vi "STED Control V4.vi"() -> ()   [LabVIEW 2014]
uses:
  Type Defs/Image Acquisition Parameters.ctl
  Laser Controls.ctl
  Detectors.ctl
  Stage Control.ctl
  Focus Control.ctl
  FPGA-7842R-Reference.ctl
  Scan Parameters.ctl
  Manual Controls V2.ctl
  XY_Stage/StageStates.ctl
  <vilib>/Utility/miscctls.llb/LVRectTypeDef.ctl
panel:
  in  "Tab Control":T1(tab)
  in  "SLM":bool
  in  "Timing":bool
  in  "Focus Control":T2
  in  "Stage Control":T3={"Halt"=FALSE, "Home"=FALSE, "Down Stage"=FALSE, "Right Stage"=FALSE, "Up Stage"=FALSE, "Left Stage"=FALSE, "Mode"=enum."Joystick", "X Position"=1.0, "Y Position"=1.0, "Step Size (um)"=enum."1", "Velocity"=enum."Low"} {"Y Position" min=1.0 max=24.0; "X Position" min=1.0 max=24.0}
  out "Channel 6":sgl[][](graph)
  out "Channel 5":sgl[][](graph)
  out "Channel 4":sgl[][](graph)
  out "Channel 3":sgl[][](graph)
  out "Channel 2":sgl[][](graph)
  in  "Dual Screens":bool=TRUE
  in  "Detectors":T4
  in  "Laser Controls":T5 {"590 Power (V)" scale=0.0..3.0; "STED Power (V)" scale=0.0..5.0}
  in  "Save File Path":path
  in  "Capture":bool
  out "Channel 1":sgl[][](graph)
  in  "Image Acquisition Parameters":T6={"Scan Type"=enum."Beam Scanning", "Scan Mode"=enum."XY", "Fast Axis Frequency (Hz)"=16110.0, "Image Format"=256, "Line Accumulations"=100, "Frames Per Capture"=1, "Frames Accumulations"=1, "Image Dimension (um)"=[15.0, 15.0], "Number of Z Steps"=1, "Z Steps Size (um)"=1.0, "Pixel Size (nm)"=[58.59375, 58.59375]} {"Z Steps Size (um)" min=0.0; "Number of Z Steps" min=1; "Frames Accumulations" min=1; "Frames Per Capture" min=1; "Line Accumulations" min=1; "Image Format" items=["64 x 64"=64, "128 x 128"=128, "256 x 256"=256, "512 x 512"=512, "1024 x 1024"=1024, "2048 x 2048"=2048]}
  in  "Live":bool
  in  "Exit":bool
  # "XY"
  # "Z"
  # "Length"
  # "Height"
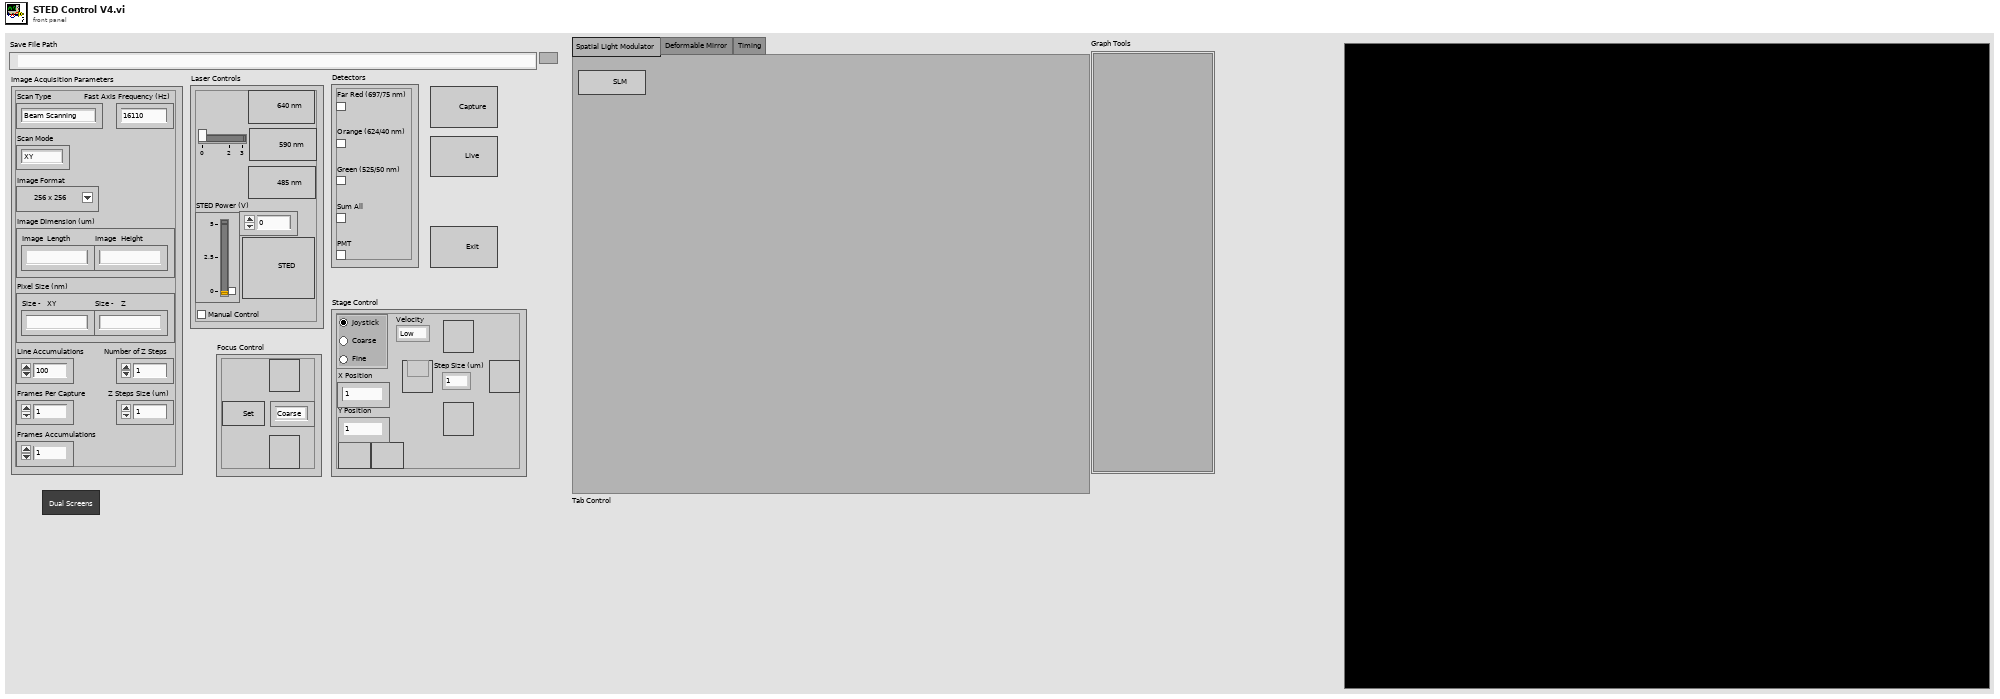
[diagram p1: front panel]
types:
  T1 = enum32{"Spatial Light Modulator", "Deformable Mirror", "Timing"}
  T2 = typedef "Focus Control.ctl" = cluster{"ZoomUp":bool, "ZoomDown":bool, "ZoomStepI16":enum16{"Coarse", "Medium", "Fine"}, "SetZoom":bool}
  T3 = typedef "Stage Control.ctl" = cluster{"Halt":bool, "Home":bool, "Down Stage":bool, "Right Stage":bool, "Up Stage":bool, "Left Stage":bool, "Mode":enum32{"Joystick", "Coarse", "Fine"}, "X Position":dbl, "Y Position":dbl, "Step Size (um)":enum16{"1", "2", "5", "10", "15", "20", "50", "100", "500"}, "Velocity":enum16{"Low", "Medium", "High"}}
  T4 = typedef "Detectors.ctl" = cluster{"PMT":bool, "Far Red (697/75 nm)":bool, "Orange (624/40 nm)":bool, "Green (525/50 nm)":bool, "Sum All":bool}
  T5 = typedef "Laser Controls.ctl" = cluster{"STED Power (V)":dbl, "590 Power (V)":dbl, "STED":bool, "640 nm":bool, "590 nm":bool, "485 nm":bool, "Manual Control":bool}
  T6 = typedef "Image Acquisition Parameters.ctl" = cluster{"Scan Type":enum16{"Sample Scanning", "Beam Scanning"}, "Scan Mode":enum16{"XY", "XZ", "YZ", "XYZ"}, "Fast Axis Frequency (Hz)":dbl, "Image Format":u16, "Line Accumulations":u16, "Frames Per Capture":u16, "Frames Accumulations":u16, "Image Dimension (um)":dbl[], "Number of Z Steps":u8, "Z Steps Size (um)":dbl, "Pixel Size (nm)":dbl[]}
  T7 = typedef "Manual Controls V2.ctl" = cluster{"Galvo 1 Position (I16)":i16, "Galvo 2 Position (I16)":i16, "X Axis Voltage (I16)":i16, "Y Axis Voltage (I16)":i16, "Z Axis Voltage (I16)":i16, "Res Mirror Amp (I16)":i16, "Res Mirror Mute":bool}
  T8 = typedef "Scan Parameters.ctl" = cluster{"Fast_Ax_Amp_V":dbl, "Fast_Ax_Off_V":dbl, "Slow_Ax_Amp_V":dbl, "Slow_Ax_Off_V ":dbl, "Slow_Ax_Max_V_VperS":dbl, "Slow_Ax1_Del25ns":i32, "Slow_Ax2_Del25ns":i32, "Stage_X_Off_V":dbl, "Stage_Y_Off_V":dbl, "Stage_Z_Off_V":dbl, "Galvo1_Off_V":dbl, "Galvo2_Off_V":dbl, "Last_Scan_Mode":enum16{"XY", "XZ", "YZ", "XYZ"}, "Current_Scan_Mode":enum16{"XY", "XZ", "YZ", "XYZ"}, "Fly_Back_Lines":u16, "Linear_Ramp_End":u32, "Z_Step_I16":i16, "Z_Start_I16":i16, "Laser_States _U32":u32, "590_Voltage_I16":i16, "775_AOM_Volt_I16":i16, "Blanking OFF":bool, "Unused_Axis_I16":i16}
  T9 = typedef "FPGA-7842R-Reference.ctl" = enum16{"Stage Control", "Laser Control", "Unused Axis I16", "Exit", "Set Res Mirror", "Set Galvo", "Default", "Close FPGA", "Stop Waveforms", "Start Waveforms", "Initialize"}
  T10 = typedef "StageStates.ctl" = enum16{"POSITION", "MVR", "MOVE", "HALT", "ONTARGET", "ERROR", "EXIT", "HOME", "ZEROPOS", "NANOPOS", "QUIT", "SERVO", "JOYSTICK", "ANALOG"}
  T11 = typedef "LVRectTypeDef.ctl" = cluster{"Left":i16, "Top":i16, "Right":i16, "Bottom":i16}
  T12 = enum32{"Invalid", "Standard", "Closed", "Hidden", "Minimized", "Maximized"}
  T13 = cluster{"Halt":bool, "Home":bool, "Down Stage":bool, "Right Stage":bool, "Up Stage":bool, "Left Stage":bool, "Mode":bool, "X Position":bool, "Y Position":bool, "Step Size (um)":bool, "Velocity":bool}
  T14 = enum16{"1", "2", "5", "10", "15", "20", "50", "100", "500"}
  T15 = typedef "Scanning Conversions.ctl" = cluster{"Stage X Axis (Volts/um)":dbl, "Stage Y Axis (Volts/um)":dbl, "Stage Z Axis (Volts/um)":dbl}
  T16 = typedef "LVAllMonitorsDisplayTypeDef.ctl" = cluster{"Bounds":cluster{"Left":i16, "Top":i16, "Right":i16, "Bottom":i16}, "Depth":i16}[]
  T17 = cluster{"Bounds":cluster{"Left":i16, "Top":i16, "Right":i16, "Bottom":i16}, "Depth":i16}
  T18 = cluster{"Scan Type":bool, "Scan Mode":bool, "Fast Axis Frequency (Hz)":bool, "Image Format":bool, "Line Accumulations":bool, "Frames Per Capture":bool, "Frames Accumulations":bool, "Image Dimension (um)":bool[], "Number of Z Steps":bool, "Z Steps Size (um)":bool, "Pixel Size (nm)":bool[]}
  T19 = typedef "IMAQ Image.ctl" = refnum<image>
  T20 = typedef "Waveform Data.ctl" = cluster{"Waveform Scan Parameters":cluster{"Scanning Mode":u8, "Fast Axis WF Length (Elements)":i32, "Fast Axis Sample Period (Ticks)":u32, "Slow Axis 1 WF Length (Elements)":i32, "Slow Axis 1 Sample Period (Ticks)":u32, "Slow Axis 1 Delay (25 ns) Steps":i32, "Slow Axis 2 WFLength (Elements)":i32, "Slow Axis 2 Sample Period (Ticks)":u32, "Slow Axis 2 Delay (25 ns) Steps":i32}, "Fast Axis Waveform":dbl[], "Slow Axis 1 Waveform":dbl[], "Slow Axis 2 Waveform":dbl[]}
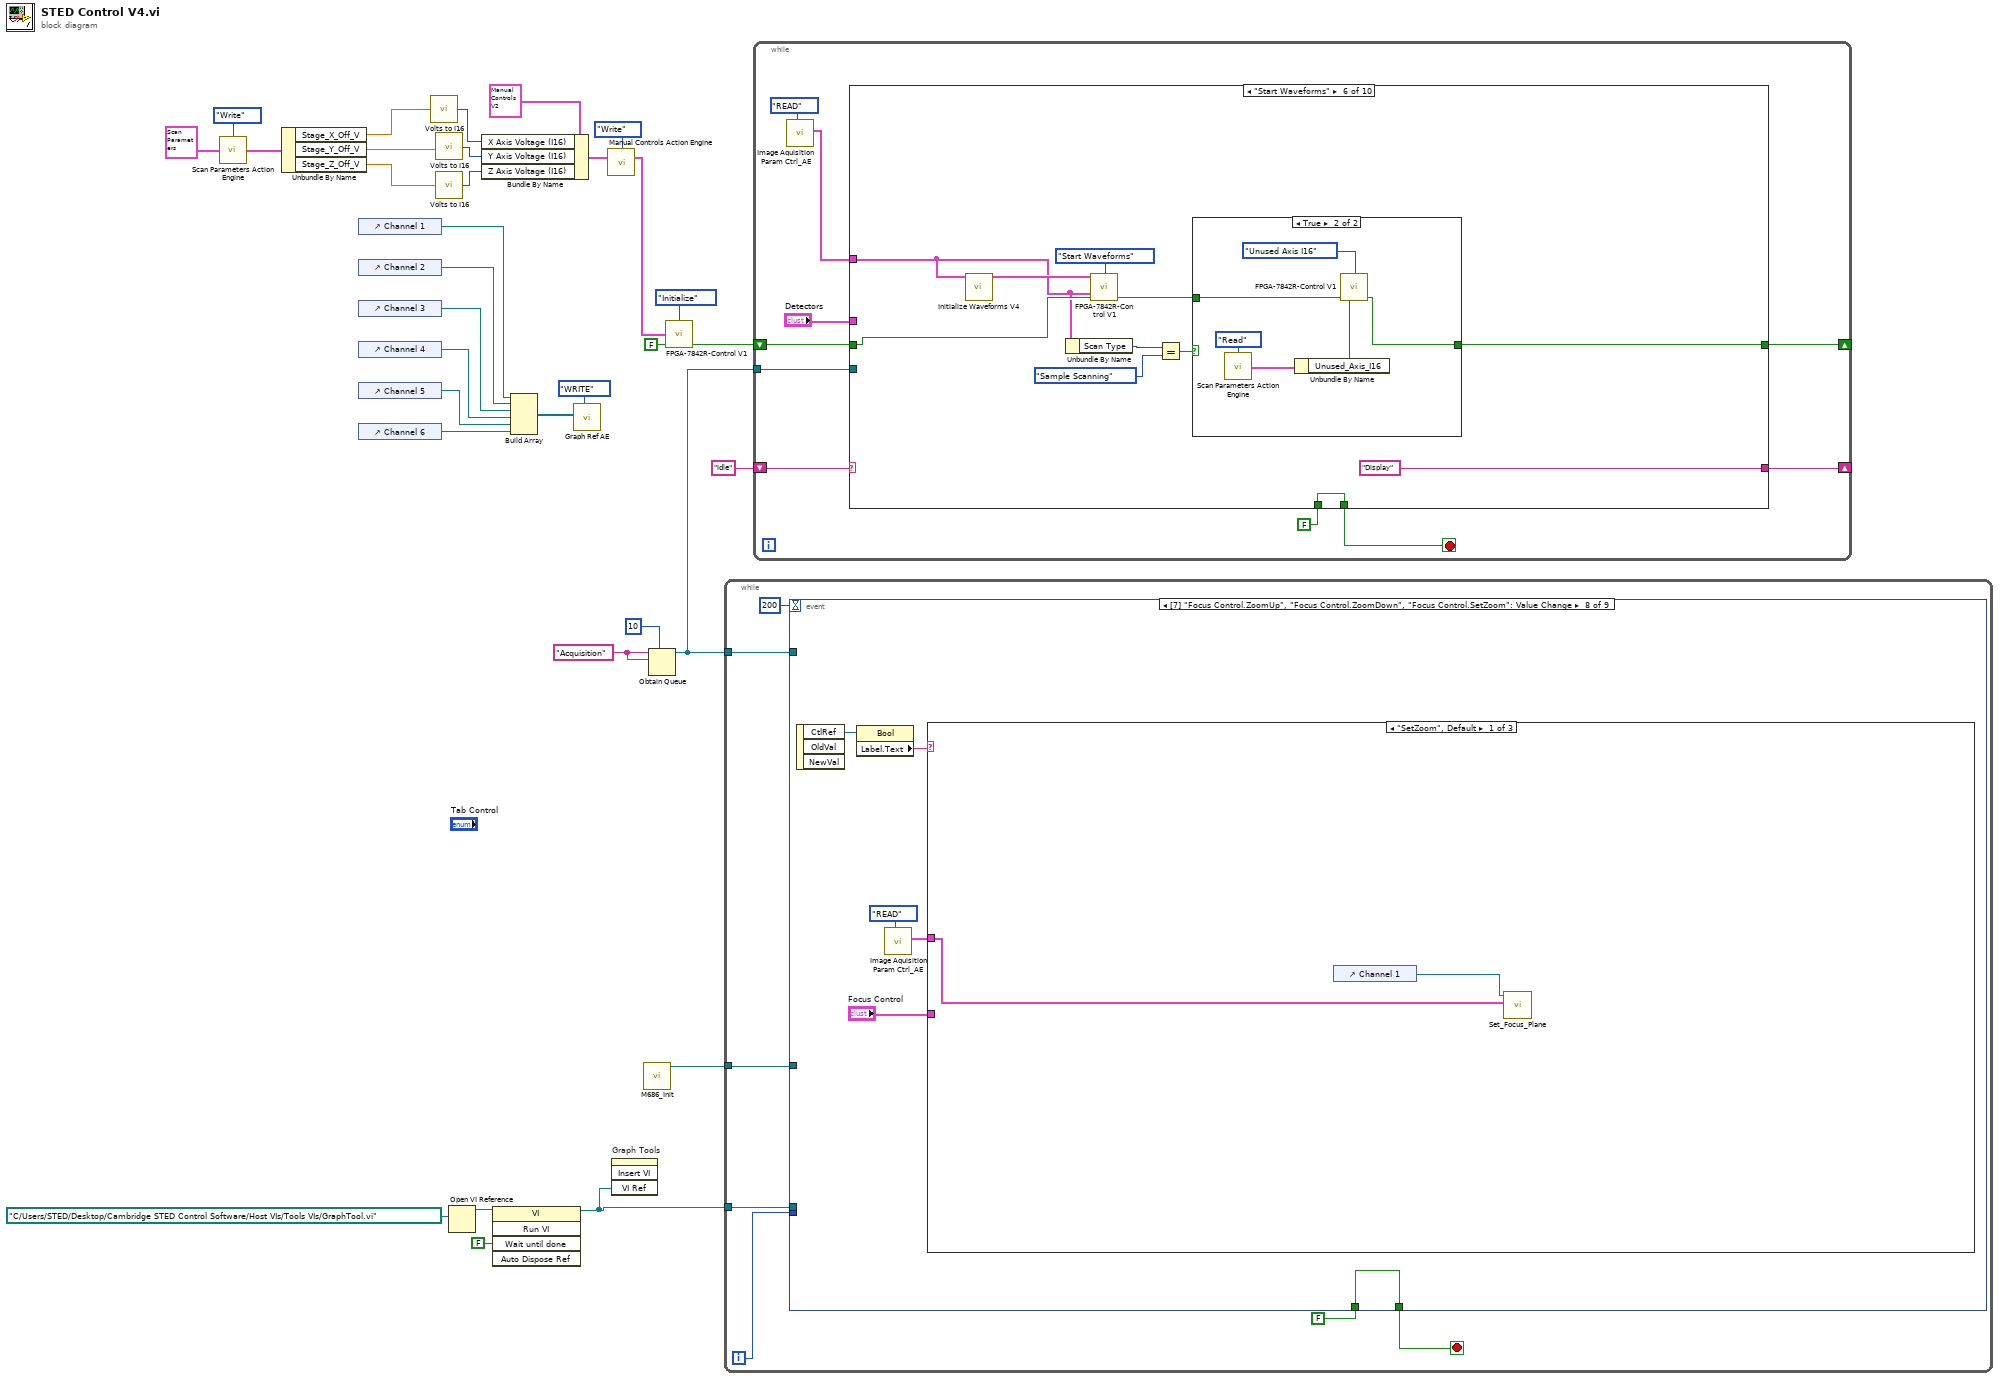
[diagram p0: block diagram]
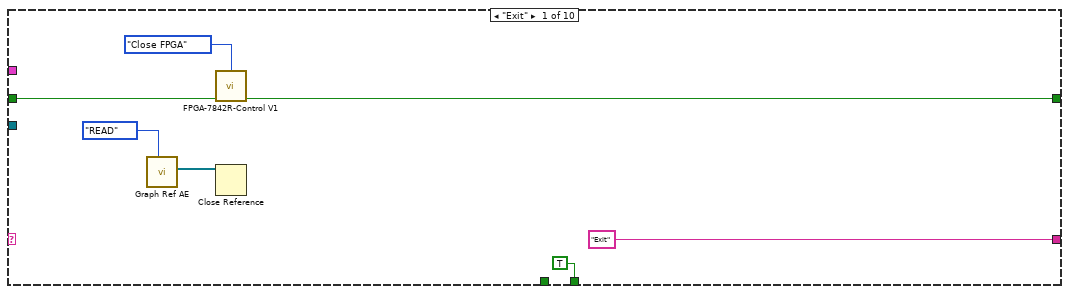
[diagram p2: hidden frame]
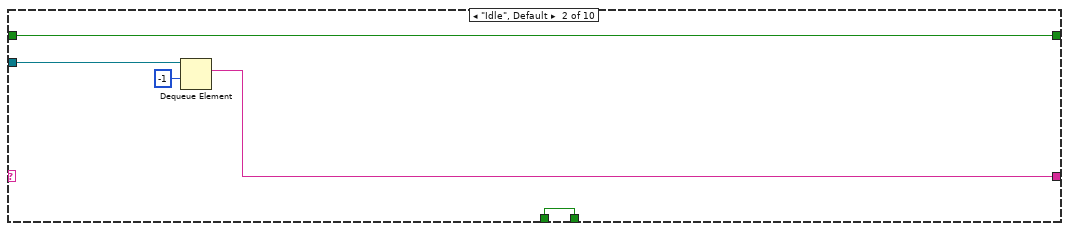
[diagram p3: hidden frame]
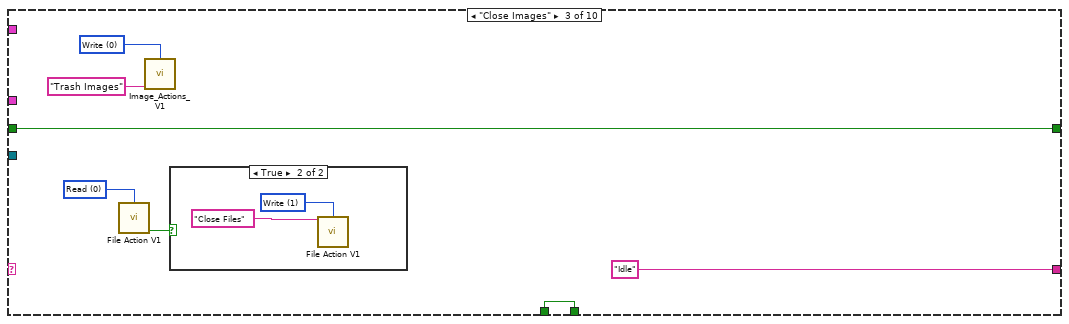
[diagram p4: hidden frame]
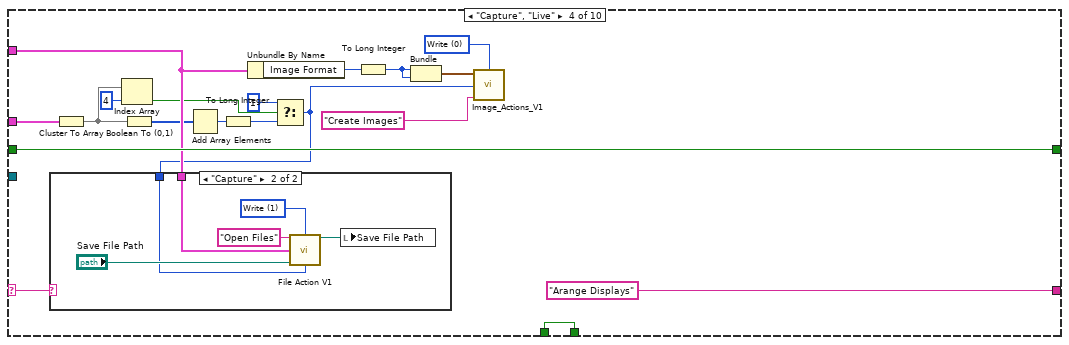
[diagram p6: hidden frame]
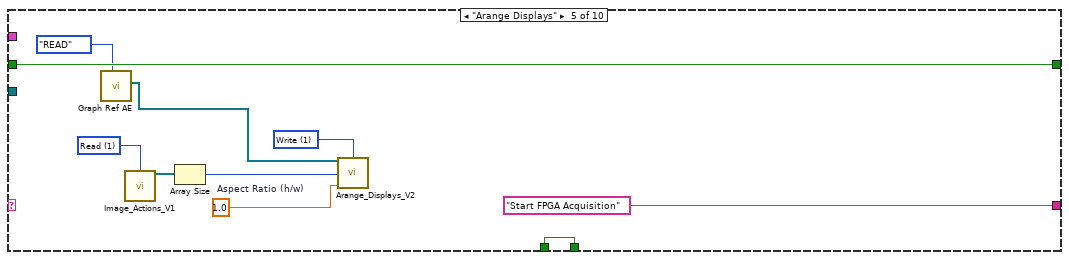
[diagram p8: hidden frame]
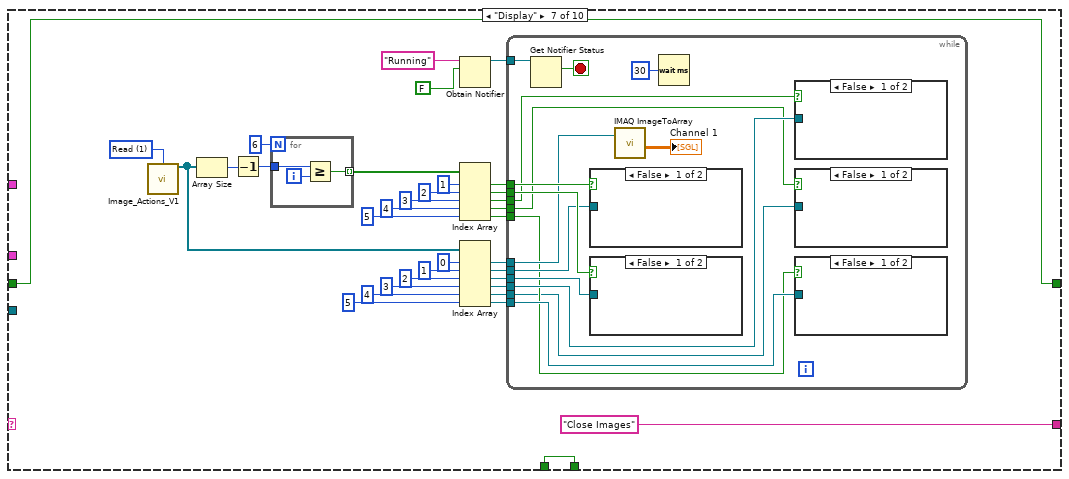
[diagram p10: hidden frame]
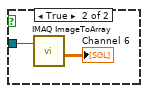
[diagram p11: hidden frame]
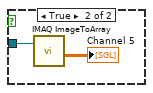
[diagram p12: hidden frame]
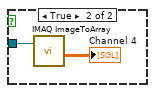
[diagram p13: hidden frame]
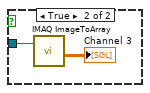
[diagram p14: hidden frame]
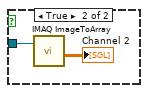
[diagram p15: hidden frame]
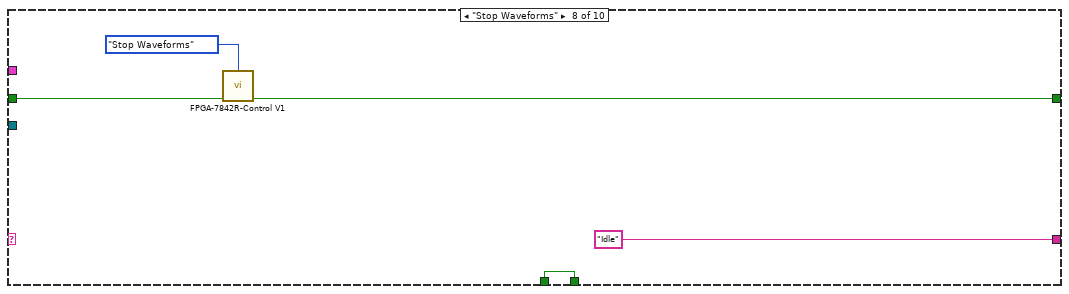
[diagram p16: hidden frame]
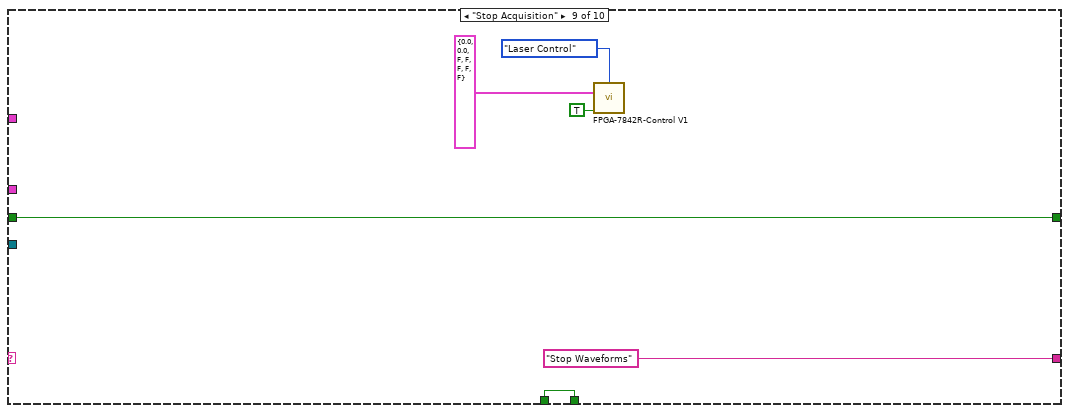
[diagram p17: hidden frame]
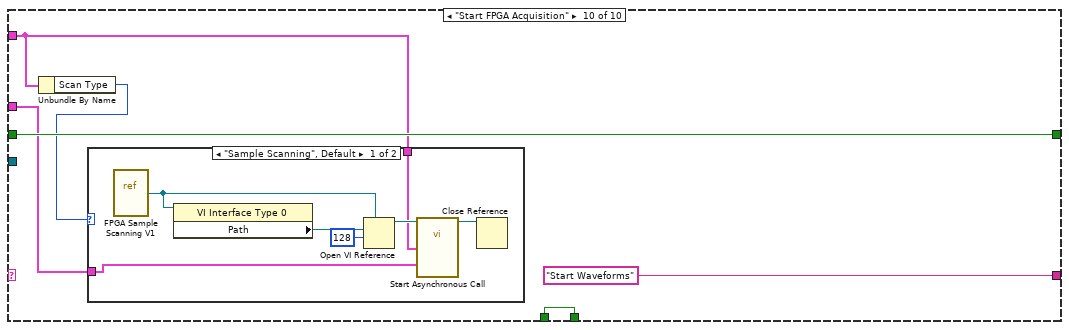
[diagram p18: hidden frame]
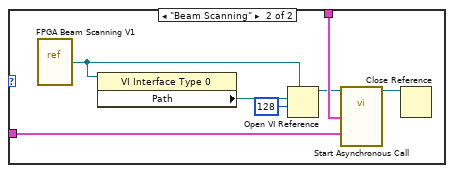
[diagram p19: hidden frame]
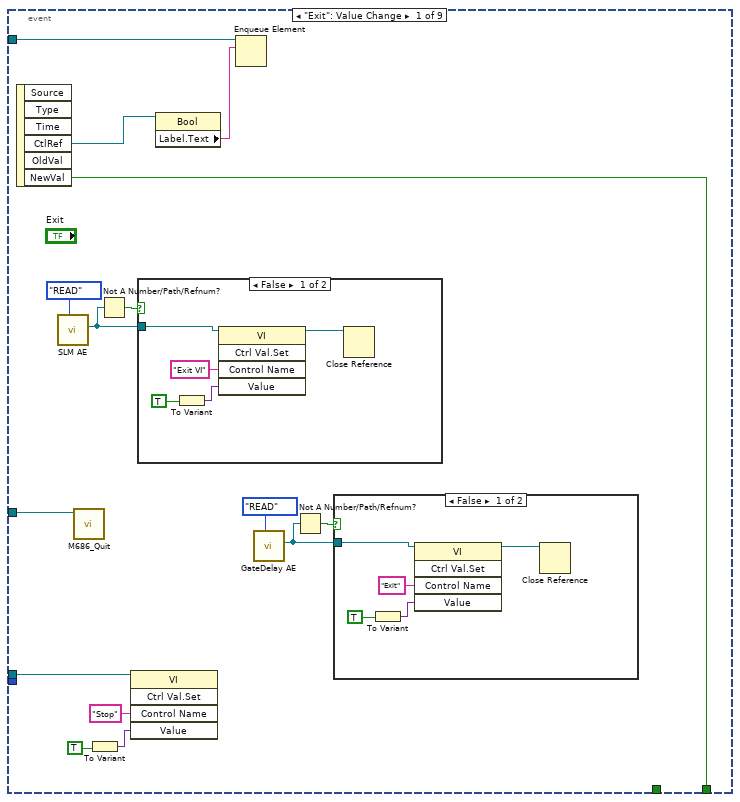
[diagram p20: hidden frame]
diagram:
  w32 = "Acquisition" ("name (unnamed)")
  n1 = call "Scan Parameters Action Engine.vi"("Action"=enum16{"Read", "Write"}."Write", "Scan Parameters IN"=T8 {"Fast_Ax_Amp_V"=0.0, "Fast_Ax_Off_V"=0.0, "Slow_Ax_Amp_V"=0.0, "Slow_Ax_Off_V "=0.0, "Slow_Ax_Max_V_VperS"=0.0, "Slow_Ax1_Del25ns"=0, "Slow_Ax2_Del25ns"=0, "Stage_X_Off_V"=5.0, "Stage_Y_Off_V"=5.0, "Stage_Z_Off_V"=5.0, "Galvo1_Off_V"=0.0, "Galvo2_Off_V"=0.0, "Last_Scan_Mode"=enum."XY", "Current_Scan_Mode"=enum."XY", "Fly_Back_Lines"=0, "Linear_Ramp_End"=0, "Z_Step_I16"=0, "Z_Start_I16"=0, "Laser_States _U32"=0, "590_Voltage_I16"=0, "775_AOM_Volt_I16"=0, "Blanking OFF"=FALSE, "Unused_Axis_I16"=16384}) -> ("Scan Parameters OUT"=w15:T8)  [unwired: 13 in]
  n2 = Unbundle By Name(w15) -> ("Stage_X_Off_V"=w11:dbl, "Stage_Y_Off_V"=w10:dbl, "Stage_Z_Off_V"=w9:dbl)
  n3 = control-ref of="Channel 1"() -> (w7:refnum<vi>)
  n4 = control-ref of="Channel 2"() -> (w24:refnum<vi>)
  n5 = control-ref of="Channel 3"() -> (w8:refnum<vi>)
  n6 = control-ref of="Channel 4"() -> (w23:refnum<vi>)
  n7 = control-ref of="Channel 5"() -> (w22:refnum<vi>)
  n8 = control-ref of="Channel 6"() -> (w21:refnum<vi>)
  n9 = call "Volts to I16.vi"("Voltage (V)"=w11) -> ("I16"=w12:i16)  [unwired: 13 in, 1 out]
  n10 = call "Volts to I16.vi"("Voltage (V)"=w10) -> ("I16"=w13:i16)  [unwired: 13 in, 1 out]
  n11 = call "Volts to I16.vi"("Voltage (V)"=w9) -> ("I16"=w14:i16)  [unwired: 13 in, 1 out]
  n12 = Open VI Reference(vi path=path "C:/Users/STED/Desktop/Cambridge STED Control Software/Host VIs/Tools VIs/GraphTool.vi") -> (vi reference=w2:refnum<vi>)  [unwired: 5 in, 1 out]
  n13 = Bundle By Name(cluster=T7 {"Galvo 1 Position (I16)"=-280, "Galvo 2 Position (I16)"=0, "X Axis Voltage (I16)"=16384, "Y Axis Voltage (I16)"=16384, "Z Axis Voltage (I16)"=16384, "Res Mirror Amp (I16)"=0, "Res Mirror Mute"=FALSE} ("Manual Controls"), "X Axis Voltage (I16)"=w12, "Y Axis Voltage (I16)"=w13, "Z Axis Voltage (I16)"=w14) -> (w16:T7)
  n14 = invoke class="VI" method="Run VI"(reference=w2, "Wait until done"=FALSE ("Wait Until Done")) -> (reference out=w4:refnum<vi>)  [unwired: 3 in, 4 out]
  n15 = Build Array(w7, w24, w8, w23, w22, w21) -> (w5:refnum<vi>[])
  n16 = call "Graph Ref AE.vi"("Action"=enum16{"READ", "WRITE"}."WRITE", "Graph Ref In"=w5) -> ()  [unwired: 9 in, 1 out]
  n17 = call "Manual Controls Action Engine.vi"("Action"=enum16{"Read", "Write"}."Write", "Manual Controls In"=w16) -> ("Manual Controls Out"=w18:T7)  [unwired: 13 in]
  n18 = invoke on="Graph Tools" class="SubPanel" method="Insert VI"("VI Ref"=w4) -> ()  [unwired: 3 in, 4 out]
  n19 = call "M686_Init.vi"() -> ("VISA Refnum out"=w20:refnum<visa-resource-name>)  [unwired: 9 in, 2 out]
  n20 = Obtain Queue(max queue size (-1, unlimited)=10, name (unnamed)=w32, element data type=w32) -> (queue out=w30:refnum<queue>)  [unwired: 2 in, 2 out]
  n21 = call "FPGA-7842R-Control V1.vi"("Action"=FPGA-7842R-Reference."Initialize", "Manual Controls"=w18, "Initialize"=FALSE) -> ("Initalized"=w27:bool)  [unwired: 12 in]
  n22 = while {
    tunnel: w30 -> [w38]
    tunnel: w20 -> [w36]
    tunnel: w4 -> [w34]
    i -> [w35]
    stop <- w40 stop-if-true
    n23 = event shown="[7] \"Focus Control.ZoomUp\", \"Focus Control.ZoomDown\", \"Focus Control.SetZoom\": Value Change" {
      selector: _ -> [_ _ _ _ _ _ _ _ _]
      dyn-events: _ -> [_ _ _ _ _ _ _ _ _]
      timeout: 200 -> [_ _ _ _ _ _ _ _ _]
      tunnel: [w55 w77 w87 w113 w280 w307 w373 w539 w645] -> w40
      tunnel: FALSE -> [_ w77 w87 w113 w280 w307 w373 w539 w645]
      tunnel: w38 -> [w54 w76 w81 _ _ _ _ _ _]
      tunnel: w36 -> [w51 _ _ w99 _ _ _ _ _]
      tunnel: w35 -> [_ _ w79 _ _ _ _ _ _]
      tunnel: w34 -> [w50 _ _ _ _ _ _ _ _]
      event "Exit": Value Change {
        n24 = event-data() -> ("CtlRef"=w53:refnum<vi>, "NewVal"=w55:bool)  [unwired: 1 in, 4 out]
        n25 = call "SLM AE.vi"("Action"=enum16{"READ", "WRITE"}."READ") -> ("SLM Ref Out"=w44:refnum<vi>)  [unwired: 10 in]
        n26 = call "M686_Quit.vi"("VISA Refnum in"=w51) -> ()  [unwired: 11 in]
        n27 = To Variant(anything=TRUE) -> (Variant=w47:variant)
        n28 = Not A Number/Path/Refnum?(number/path/refnum=w44) -> (NaN/Path/Refnum?=w45:bool)
        n29 = invoke class="VI" method="Ctrl Val.Set"(reference=w50, "Control Name"="Stop", "Value"=w47) -> ()  [unwired: 2 in, 5 out]
        n30 = case shown="False" w45 {
          tunnel: w44 -> [w61 _]
          frame False {
            n31 = To Variant(anything=TRUE) -> (Variant=w62:variant)
            n32 = invoke class="VI" method="Ctrl Val.Set"(reference=w61, "Control Name"="Exit VI", "Value"=w62) -> (reference out=w65:refnum<vi>)  [unwired: 2 in, 4 out]
            n33 = Close Reference(reference=w65) -> ()  [unwired: 1 in, 1 out]
          }
          frame True {
          }
        }
        n34 = property class="Bool"(reference=w53) -> ("Label.Text"=w52:string)  [unwired: 1 in, 2 out]
        n35 = Enqueue Element(queue=w54, element=w52) -> ()  [unwired: 2 in, 3 out]
        n36 = call "GateDelay AE.vi"("Action"=enum16{"READ", "WRITE"}."READ") -> ("Gate Delay Ref Out"=w43:refnum<vi>)  [unwired: 10 in]
        n37 = Not A Number/Path/Refnum?(number/path/refnum=w43) -> (NaN/Path/Refnum?=w42:bool)
        n38 = case shown="False" w42 {
          tunnel: w43 -> [w56 _]
          frame False {
            n39 = To Variant(anything=TRUE) -> (Variant=w57:variant)
            n40 = invoke class="VI" method="Ctrl Val.Set"(reference=w56, "Control Name"="Exit", "Value"=w57) -> (reference out=w60:refnum<vi>)  [unwired: 2 in, 4 out]
            n41 = Close Reference(reference=w60) -> ()  [unwired: 1 in, 1 out]
          }
          frame True {
          }
        }
      }
      event "Live", "Capture": Value Change {
        n42 = event-data() -> ("CtlRef"=w75:refnum<vi>, "NewVal"=w67:bool)  [unwired: 1 in]
        n43 = property on="Channel 1" class="IntGraph (strict)"("Cursor.Visible"=FALSE) -> ()  [unwired: 2 in, 2 out]
        n44 = property class="Bool (strict)"(reference=w75) -> ("Label.Text"=w66:string)  [unwired: 1 in, 2 out]
        n45 = Obtain Notifier(name (unnamed)="Running", notification data type=TRUE) -> (notifier out=w72:refnum<notifier>)  [unwired: 2 in, 2 out]
        n46 = Not(x=w67) -> (.not. x?=w70:bool)
        n47 = Send Notification(notification=w70, notifier=w72) -> ()  [unwired: 1 in, 2 out]
        n48 = Select(t=w66, s=w67, f="Stop Acquisition") -> (s? t:f=w68:string)
        n49 = Enqueue Element(queue=w76, element=w68) -> ()  [unwired: 2 in, 3 out]
      }
      event Timeout {
        n50 = event-data() -> ()  [unwired: 1 in, 3 out]
        n51 = Equal To 0?(x=w79) -> (x = 0?=w78:bool)
        n52 = case shown="False" w78 {
          frame False {
            n53 = call "Image Aquisition Param Ctrl_AE.vi"("Action"=enum16{"READ", "WRITE"}."READ") -> ("Image Acquisition Parameters Out"=w89:T6)  [unwired: 10 in]
            n54 = local write "Image Acquisition Parameters"(w89) -> ()
          }
          frame True {
            n55 = local read "Image Acquisition Parameters"() -> (w90:T6)
            n56 = call "Image Aquisition Param Ctrl_AE.vi"("Action"=enum16{"READ", "WRITE"}."WRITE", "Image Acquisition Parameters In"=w90) -> ()  [unwired: 9 in, 1 out]
          }
        }
        n57 = Obtain Notifier(name (unnamed)="Running", notification data type=TRUE) -> (notifier out=w85:refnum<notifier>)  [unwired: 2 in, 2 out]
        n58 = Get Notifier Status(notifier=w85) -> (current notification=w83:bool)  [unwired: 1 in, 4 out]
        n59 = local read "Capture"() -> (w82:bool)
        n60 = And(x=w83, y=w82) -> (x .and. y?=w80:bool)
        n61 = case shown="False" w80 {
          tunnel: w81 -> [_ w93]
          frame False {
          }
          frame True {
            n62 = local write "Capture"(FALSE ("Capture")) -> ()
            n63 = Enqueue Element(queue=w93, element="Stop Acquisition" ("f")) -> ()  [unwired: 2 in, 3 out]
          }
        }
      }
      event Value Change {
        n64 = event-data() -> ("OldVal"=w115:T3, "NewVal"=w114:T3)  [unwired: 1 in, 4 out]
        n65 = property on="Stage Control" class="Clust"() -> ("Controls[]"=w101:refnum<vi>[])  [unwired: 2 in, 2 out]
        n66 = Not Equal?(x=w115, y=w114) -> (x != y?=w100:T13)
        n67 = Unbundle By Name(w114) -> ("Mode"=w107:enum32{"Joystick", "Coarse", "Fine"}, "Step Size (um)"=w106:T14, "Velocity"=w104:enum16{"Low", "Medium", "High"})
        n68 = Cluster To Array(cluster=w100) -> (array=w109:bool[])
        n69 = for {
          tunnel: w101 -> [w274] mode=indexing
          tunnel: w109 -> [w275] mode=indexing
          tunnel: [w274] -> w110
          stop <- w275 stop-if-true
        }
        n70 = Format Into String(w104) -> (resulting string=w103:string)  [unwired: 3 in, 1 out]
        n71 = Format Into String(w106) -> (resulting string=w108:string)  [unwired: 3 in, 1 out]
        n72 = case shown="\"Medium\", Default" w103 {
          tunnel: [0.5 1.0 0.1] -> w102
          frame "Medium", Default {
          }
          frame "High" {
          }
          frame "Low" {
          }
        }
        n73 = property class="Ctl"(reference=w110) -> ("ClassName"=w111:string, "Label.Text"=w112:string)  [unwired: 1 in, 2 out]
        n74 = control-ref of="Halt"() -> (w97:refnum<vi>)
        n75 = Fract/Exp String To Number(string=w108) -> (number=w105:dbl)  [unwired: 3 in, 1 out]
        n76 = case shown="\"Coarse\"" w107 {
          tunnel: w99 -> [w124 w137 w208 w219]
          tunnel: w111 -> [_ w136 _ w218]
          tunnel: w112 -> [_ w135 _ w217]
          tunnel: [w123 w134 w207 w216] -> w98
          tunnel: w97 -> [w122 w133 w206 w214]
          tunnel: w105 -> [_ w132 _ w215]
          tunnel: w102 -> [w121 w131 _ _]
          frame "Joystick" {
            w119 = TRUE
            n77 = Build Array(w119, w119) -> (w118:bool[])
            n78 = call "M686.vi"("Velocity"=w121, "Abort"=w122, "Axis"=w118, "Action"=StageStates."JOYSTICK", "VISA In"=w124) -> ("VISA Out"=w117:refnum<visa-resource-name>)  [unwired: 3 in, 3 out]
            n79 = call "M686.vi"("Abort"=w122, "Action"=StageStates."POSITION", "VISA In"=w117) -> ("Position Out"=w123:dbl[])  [unwired: 5 in, 3 out]
          }
          frame "Coarse" {
            w129 = FALSE
            n80 = Build Array(w129, w129) -> (w128:bool[])
            n81 = call "M686.vi"("Abort"=w133, "Axis"=w128, "Action"=StageStates."JOYSTICK", "VISA In"=w137) -> ("VISA Out"=w127:refnum<visa-resource-name>)  [unwired: 4 in, 3 out]
            n82 = Divide(x=w132, y=1000.0) -> (x/y=w126:dbl)
            n83 = case shown="\"Boolean\"" w136 {
              tunnel: w135 -> [_ w147]
              tunnel: w127 -> [w141 w146]
              tunnel: w126 -> [_ w145]
              tunnel: w133 -> [w138 w144]
              tunnel: [w140 w143] -> w134
              tunnel: w131 -> [_ w142]
              frame Default {
                n84 = call "M686.vi"("Abort"=w138, "Action"=StageStates."POSITION", "VISA In"=w141) -> ("Position Out"=w140:dbl[])  [unwired: 5 in, 3 out]
              }
              frame "Boolean" {
                n85 = case shown="\"Right Stage\"" w147 {
                  tunnel: w146 -> [_ w152 w162 w170 w183 w193 w204]
                  tunnel: w145 -> [_ _ _ w169 w182 w184 w203]
                  tunnel: w144 -> [_ w150 w161 w171 w181 w192 w202]
                  tunnel: [dbl[] [] ("Position Out") w149 w160 w172 w180 w191 w201] -> w143
                  tunnel: w142 -> [_ _ _ w168 w179 w190 w200]
                  frame Default {
                  }
                  frame "Home" {
                    w154 = TRUE
                    n86 = Build Array(w154, w154) -> (w155:bool[])
                    n87 = call "M686.vi"("Velocity"=1.0, "Abort"=w150, "Axis"=w155, "Action"=StageStates."HOME", "VISA In"=w152) -> ("Position Out"=w149:dbl[])  [unwired: 3 in, 3 out]
                  }
                  frame "Halt" {
                    w158 = TRUE
                    n88 = Build Array(w158, w158) -> (w159:bool[])
                    n89 = call "M686.vi"("Velocity"=1.0, "Abort"=w161, "Axis"=w159, "Action"=StageStates."HALT", "VISA In"=w162) -> ("Position Out"=w160:dbl[])  [unwired: 3 in, 3 out]
                  }
                  frame "Up Stage" {
                    n90 = Build Array(w169, w169) -> (w166:dbl[])
                    n91 = Build Array(FALSE, TRUE) -> (w163:bool[])
                    n92 = call "M686.vi"("Velocity"=w168, "Abort"=w171, "Axis"=w163, "Positions"=w166, "Action"=StageStates."MVR", "VISA In"=w170) -> ("Position Out"=w172:dbl[])  [unwired: 2 in, 3 out]
                  }
                  frame "Down Stage" {
                    n93 = Negate(x=w182) -> (-x=w173:dbl)
                    n94 = Build Array(w173, w173) -> (w177:dbl[])
                    n95 = Build Array(FALSE, TRUE) -> (w174:bool[])
                    n96 = call "M686.vi"("Velocity"=w179, "Abort"=w181, "Axis"=w174, "Positions"=w177, "Action"=StageStates."MVR", "VISA In"=w183) -> ("Position Out"=w180:dbl[])  [unwired: 2 in, 3 out]
                  }
                  frame "Left Stage" {
                    n97 = Build Array(w184, w184) -> (w188:dbl[])
                    n98 = Build Array(TRUE, FALSE) -> (w185:bool[])
                    n99 = call "M686.vi"("Velocity"=w190, "Abort"=w192, "Axis"=w185, "Positions"=w188, "Action"=StageStates."MVR", "VISA In"=w193) -> ("Position Out"=w191:dbl[])  [unwired: 2 in, 3 out]
                  }
                  frame "Right Stage" {
                    n100 = Negate(x=w203) -> (-x=w194:dbl)
                    n101 = Build Array(w194, w194) -> (w198:dbl[])
                    n102 = Build Array(TRUE, FALSE) -> (w195:bool[])
                    n103 = call "M686.vi"("Velocity"=w200, "Abort"=w202, "Axis"=w195, "Positions"=w198, "Action"=StageStates."MVR", "VISA In"=w204) -> ("Position Out"=w201:dbl[])  [unwired: 2 in, 3 out]
                  }
                }
              }
            }
          }
          frame Default {
            n104 = call "M686.vi"("Abort"=w206, "Action"=StageStates."POSITION", "VISA In"=w208) -> ("Position Out"=w207:dbl[])  [unwired: 5 in, 3 out]
          }
          frame "Fine" {
            w212 = FALSE
            n105 = case shown="\"Boolean\"" w218 {
              tunnel: w217 -> [_ w229]
              tunnel: w215 -> [_ w228]
              frame "False", Default {
              }
              frame "Boolean" {
                n106 = call "Manual Controls Action Engine.vi"("Action"=enum16{"Read", "Write"}."Read") -> ("Manual Controls Out"=w226:T7)  [unwired: 14 in]
                n107 = call "Scanning Volts to Microns.vi"() -> ("Scanning Conversions OUT"=w227:T15)
                n108 = case shown="Default" w229 {
                  tunnel: w228 -> [_ w238 _ w251 w260 w269]
                  tunnel: w227 -> [_ w239 _ w252 w261 w270]
                  tunnel: w226 -> [w230 w237 w243 w250 w259 w268]
                  tunnel: [w230 w236 w242 w249 w258 w267] -> w224
                  frame Default {
                  }
                  frame "Up Stage" {
                    n109 = Unbundle By Name(w239) -> ("Stage Y Axis (Volts/um)"=w235:dbl)
                    n110 = Unbundle By Name(w237) -> ("Y Axis Voltage (I16)"=w234:i16)
                    n111 = Multiply(x=w238, y=w235) -> (x*y=w232:dbl)
                    n112 = call "Volts to I16.vi"("Voltage (V)"=w232) -> ("I16"=w231:i16)  [unwired: 13 in, 1 out]
                    n113 = Subtract(x=w234, y=w231) -> (x-y=w233:i16)
                    n114 = Bundle By Name(cluster=w237, "Y Axis Voltage (I16)"=w233) -> (w236:T7)
                  }
                  frame "Home" {
                    n115 = call "Volts to I16.vi"("Voltage (V)"=5.0 ("Stage Y Axis Offset (V)")) -> ("I16"=w240:i16)  [unwired: 13 in, 1 out]
                    n116 = Bundle By Name(cluster=w243, "X Axis Voltage (I16)"=w240, "Y Axis Voltage (I16)"=w240) -> (w242:T7)
                  }
                  frame "Down Stage" {
                    n117 = Unbundle By Name(w250) -> ("Y Axis Voltage (I16)"=w247:i16)
                    n118 = Unbundle By Name(w252) -> ("Stage Y Axis (Volts/um)"=w248:dbl)
                    n119 = Multiply(x=w251, y=w248) -> (x*y=w245:dbl)
                    n120 = call "Volts to I16.vi"("Voltage (V)"=w245) -> ("I16"=w244:i16)  [unwired: 13 in, 1 out]
                    n121 = Add(x=w247, y=w244) -> (x+y=w246:i16)
                    n122 = Bundle By Name(cluster=w250, "Y Axis Voltage (I16)"=w246) -> (w249:T7)
                  }
                  frame "Left Stage" {
                    n123 = Unbundle By Name(w261) -> ("Stage X Axis (Volts/um)"=w257:dbl)
                    n124 = Unbundle By Name(w259) -> ("X Axis Voltage (I16)"=w256:i16)
                    n125 = Multiply(x=w260, y=w257) -> (x*y=w254:dbl)
                    n126 = call "Volts to I16.vi"("Voltage (V)"=w254) -> ("I16"=w253:i16)  [unwired: 13 in, 1 out]
                    n127 = Subtract(x=w256, y=w253) -> (x-y=w255:i16)
                    n128 = Bundle By Name(cluster=w259, "X Axis Voltage (I16)"=w255) -> (w258:T7)
                  }
                  frame "Right Stage" {
                    n129 = Unbundle By Name(w270) -> ("Stage X Axis (Volts/um)"=w266:dbl)
                    n130 = Unbundle By Name(w268) -> ("X Axis Voltage (I16)"=w265:i16)
                    n131 = Multiply(x=w269, y=w266) -> (x*y=w263:dbl)
                    n132 = call "Volts to I16.vi"("Voltage (V)"=w263) -> ("I16"=w262:i16)  [unwired: 13 in, 1 out]
                    n133 = Add(x=w265, y=w262) -> (x+y=w264:i16)
                    n134 = Bundle By Name(cluster=w268, "X Axis Voltage (I16)"=w264) -> (w267:T7)
                  }
                }
                n135 = call "Manual Controls Action Engine.vi"("Action"=enum16{"Read", "Write"}."Write", "Manual Controls In"=w224) -> ("Manual Controls Out"=w221:T7)  [unwired: 13 in]
                n136 = call "FPGA-7842R-Control V1.vi"("Action"=FPGA-7842R-Reference."Stage Control", "Manual Controls"=w221, "Initialize"=TRUE) -> ()  [unwired: 12 in, 1 out]
              }
            }
            n137 = Build Array(w212, w212) -> (w211:bool[])
            n138 = call "M686.vi"("Abort"=w214, "Axis"=w211, "Action"=StageStates."JOYSTICK", "VISA In"=w219) -> ("VISA Out"=w210:refnum<visa-resource-name>)  [unwired: 4 in, 3 out]
            n139 = call "M686.vi"("Abort"=w214, "Action"=StageStates."POSITION", "VISA In"=w210) -> ("Position Out"=w216:dbl[])  [unwired: 5 in, 3 out]
          }
        }
        n140 = Index Array(array=w98) -> (element #1=w96:dbl, element #2=w95:dbl)  [unwired: 2 in]
        n141 = property on="X Position" class="DigNum (strict)"("Value"=w96) -> ()  [unwired: 2 in, 2 out]
        n142 = property on="Y Position" class="DigNum (strict)"("Value"=w95) -> ()  [unwired: 2 in, 2 out]
      }
      event Value Change {
        w293 = FALSE ("element")
        n143 = event-data() -> ()  [unwired: 1 in, 6 out]
        n144 = Unbundle By Name("Laser Controls") -> ("STED"=w299:bool, "640 nm"=w296:bool, "590 nm"=w297:bool, "485 nm"=w298:bool, "590 Power (V)"=w290:dbl, "STED Power (V)"=w289:dbl, "Manual Control"=w277:bool)
        n145 = Build Array(w299, w296, w297, w298, w293, w293, w293, w293) -> (w295:bool[])
        n146 = local read "Live"() -> (w278:bool)
        n147 = Boolean Array To Number(Boolean array=w295) -> (number=w294:u32)
        n148 = To Unsigned Byte Integer(number=w294) -> (unsigned 8bit integer=w292:u8)
        n149 = Or(x=w278, y=w277) -> (x .or. y?=w276:bool)
        n150 = In Range and Coerce(upper limit=3.0, x=w290, lower limit=0.0) -> (coerced(x)=w284:dbl)  [unwired: 1 out]
        n151 = In Range and Coerce(upper limit=5.0, x=w289, lower limit=0.0) -> (coerced(x)=w283:dbl)  [unwired: 1 out]
        n152 = call "U8_To_U32.vi"("U8 IN"=w292) -> ("U32 OUT"=w291:u32)  [unwired: 13 in, 1 out]
        n153 = call "Volts to I16.vi"("Voltage (V)"=w284) -> ("I16"=w282:i16)  [unwired: 13 in, 1 out]
        n154 = call "Volts to I16.vi"("Voltage (V)"=w283) -> ("I16"=w281:i16)  [unwired: 13 in, 1 out]
        n155 = case shown="True" w276 {
          tunnel: "Laser Controls" -> [_ w305]
          frame False {
          }
          frame True {
            n156 = call "FPGA-7842R-Control V1.vi"("Action"=FPGA-7842R-Reference."Laser Control", "Laser Controls"=w305, "Initialize"=TRUE) -> ()  [unwired: 12 in, 1 out]
          }
        }
        n157 = call "Scan Parameters Action Engine.vi"("Action"=enum16{"Read", "Write"}."Read") -> ("Scan Parameters OUT"=w302:T8)  [unwired: 14 in]
        n158 = Bundle By Name(cluster=w302, "Laser_States _U32"=w291, "590_Voltage_I16"=w282, "775_AOM_Volt_I16"=w281) -> (w300:T8)
        n159 = call "Scan Parameters Action Engine.vi"("Action"=enum16{"Read", "Write"}."Write", "Scan Parameters IN"=w300) -> ()  [unwired: 13 in, 1 out]
      }
      event "Dual Screens": Value Change {
        n160 = event-data() -> ("NewVal"=w309:bool)  [unwired: 1 in, 5 out]
        n161 = property class="App"() -> ("Disp.AllMonitors"=w310:T16)  [unwired: 2 in, 2 out]
        n162 = control-ref of="This VI"() -> (w308:refnum<vi>)
        n163 = case shown="False" w309 {
          tunnel: w310 -> [w313 w326]
          tunnel: T11 {"Left"=0, "Top"=0, "Right"=0, "Bottom"=0} ("FP Window Bounds 2") -> [w312 w325]
          tunnel: w308 -> [_ w324]
          frame False {
            w316 = i16 0
            n164 = Index Array(array=w313, index=0) -> (element=w320:T17)
            n165 = Unbundle By Name(w320) -> ("Bounds.Right"=w321:i16, "Bounds.Bottom"=w318:i16, "Bounds.Top"=w317:i16)
            n166 = Subtract(x=w318, y=w317) -> (x-y=w315:i16)
            n167 = Bundle By Name(cluster=w312, "Left"=w316, "Top"=w316, "Right"=w321, "Bottom"=w315) -> (w314:T11)
            n168 = property class="VI"("Front Panel.WinBounds"=w314) -> (reference out=w323:refnum<vi>)  [unwired: 2 in, 1 out]
            n169 = property class="VI"(reference=w323, "FP.State"=T12."Maximized" ("Front Panel Window:State")) -> ()  [unwired: 1 in, 2 out]
          }
          frame True {
            w335 = i16 0
            n170 = Index Array(array=w326, index #1=1 ("index"), index #2=0 ("index")) -> (element #1=w329:T17, element #2=w330:T17)
            n171 = Unbundle By Name(w329) -> ("Bounds.Right"=w331:i16)
            n172 = Unbundle By Name(w330) -> ("Bounds.Left"=w332:i16, "Bounds.Bottom"=w333:i16, "Bounds.Top"=w334:i16)
            n173 = Subtract(x=w331, y=w332) -> (x-y=w336:i16)
            n174 = Subtract(x=w333, y=w334) -> (x-y=w337:i16)
            n175 = Bundle By Name(cluster=w325, "Left"=w335, "Top"=w335, "Right"=w336, "Bottom"=w337) -> (w338:T11)
            n176 = property class="VI"(reference=w324, "Front Panel.WinBounds"=w338) -> ()  [unwired: 1 in, 2 out]
          }
        }
      }
      event Value Change {
        n177 = event-data() -> ("OldVal"=w360:T6, "NewVal"=w353:T6)  [unwired: 1 in]
        n178 = Not Equal?(x=w360, y=w353) -> (x != y?=w359:T18)
        n179 = Unbundle By Name(w359) -> ("Scan Mode"=w358:bool, "Image Dimension (um)"=w340:bool[], "Image Format"=w348:bool, "Pixel Size (nm)"=w339:bool[])
        n180 = Or Array Elements(Boolean array=w339) -> (logical OR=w352:bool)
        n181 = case shown="True" w352 {
          tunnel: w353 -> [w374 w382]
          tunnel: [w374 w380] -> w351
          tunnel: w339 -> [_ w378]
          frame False {
          }
          frame True {
            n182 = Unbundle By Name(w382) -> ("Pixel Size (nm)"=w377:dbl[], "Image Format"=w386:u16)
            n183 = for {
              tunnel: w378 -> [w387] mode=indexing
              tunnel: w377 -> [w388] mode=indexing
              tunnel: [w388] -> w379
              stop <- w387 stop-if-true
            }
            n184 = Array Size(array=w377) -> (size(s)=w376:i32)
            n185 = To Double Precision Float(number=w386) -> (double precision float=w384:dbl)
            n186 = Initialize Array(w379, w376) -> (w375:dbl[])
            n187 = Multiply(x=w375, y=w384) -> (x*y=w385:dbl[])
            n188 = Multiply(x=w385, y=0.001) -> (x*y=w381:dbl[])
            n189 = Bundle By Name(cluster=w382, "Pixel Size (nm)"=w375, "Image Dimension (um)"=w381) -> (w380:T6)
          }
        }
        n190 = Or Array Elements(Boolean array=w340) -> (logical OR=w350:bool)
        n191 = Or(x=w350, y=w348) -> (x .or. y?=w349:bool)
        n192 = case shown="False" w358 {
          tunnel: w353 -> [_ w406]
          tunnel: w360 -> [_ w408]
          frame False {
            n193 = property on="Channel 1" class="IntGraph (strict)"("Cursor.Visible"=FALSE) -> ()  [unwired: 2 in, 2 out]
          }
          frame True {
            n194 = Unbundle By Name(w406) -> ("Scan Type"=w405:enum16{"Sample Scanning", "Beam Scanning"}, "Image Format"=w409:u16, "Scan Mode"=w407:enum16{"XY", "XZ", "YZ", "XYZ"})
            n195 = case shown="\"Sample Scanning\", Default" w405 {
              tunnel: w409 -> [w421 _]
              tunnel: w408 -> [w420 _]
              tunnel: w407 -> [w413 _]
              frame "Sample Scanning", Default {
                n196 = Unbundle By Name(w420) -> ("Scan Mode"=w414:enum16{"XY", "XZ", "YZ", "XYZ"})
                n197 = call "Scan Parameters Action Engine.vi"("Action"=enum16{"Read", "Write"}."Read") -> ("Scan Parameters OUT"=w416:T8)  [unwired: 14 in]
                n198 = To Double Precision Float(number=w421) -> (double precision float=w410:dbl)
                n199 = case shown="\"XY\", Default" w414 {
                  tunnel: w410 -> [w426 w454 w482 w510]
                  tunnel: w410 -> [w425 w453 w481 w509]
                  tunnel: w413 -> [w427 w455 w483 w511]
                  tunnel: [w424 w452 w480 w508] -> w419
                  tunnel: [w423 w451 w479 w507] -> w418
                  tunnel: [w422 w450 w478 w506] -> w417
                  frame "XY", Default {
                    n200 = case shown="\"XZ\"" w427 {
                      tunnel: w426 -> [w429 w436 w441 w443]
                      tunnel: w425 -> [w430 w433 w440 w447]
                      tunnel: [w429 w432 w438 w444] -> w424
                      tunnel: [w430 w431 w437 w448] -> w423
                      tunnel: [FALSE ("Cursor.Visible") TRUE ("Cursor.Visible") TRUE ("Cursor.Visible") FALSE ("Cursor.Visible")] -> w422
                      frame "XY", Default {
                      }
                      frame "XZ" {
                        n201 = Divide(x=w436, y=2.0) -> (x/y=w431:dbl)
                        n202 = Increment(x=w433) -> (x+1=w432:dbl)
                      }
                      frame "YZ" {
                        n203 = Increment(x=w441) -> (x+1=w437:dbl)
                        n204 = Divide(x=w440, y=2.0) -> (x/y=w438:dbl)
                      }
                      frame "XYZ" {
                        n205 = Divide(x=w443, y=2.0) -> (x/y=w444:dbl)
                        n206 = Divide(x=w447, y=2.0) -> (x/y=w448:dbl)
                      }
                    }
                  }
                  frame "XZ" {
                    n207 = case shown="\"XYZ\"" w455 {
                      tunnel: w454 -> [w457 w464 w468 w471]
                      tunnel: w453 -> [w459 w463 w466 w475]
                      tunnel: [w456 w464 w465 w472] -> w452
                      tunnel: [w458 w463 w467 w476] -> w451
                      tunnel: [TRUE ("Cursor.Visible") FALSE ("Cursor.Visible") TRUE ("Cursor.Visible") FALSE ("Cursor.Visible")] -> w450
                      frame "XY" {
                        n208 = Increment(x=w457) -> (x+1=w456:dbl)
                        n209 = Divide(x=w459, y=2.0) -> (x/y=w458:dbl)
                      }
                      frame "XZ", Default {
                      }
                      frame "YZ" {
                        n210 = Increment(x=w466) -> (x+1=w467:dbl)
                        n211 = Divide(x=w468, y=2.0) -> (x/y=w465:dbl)
                      }
                      frame "XYZ" {
                        n212 = Divide(x=w471, y=2.0) -> (x/y=w472:dbl)
                        n213 = Divide(x=w475, y=2.0) -> (x/y=w476:dbl)
                      }
                    }
                  }
                  frame "YZ" {
                    n214 = case shown="\"XY\"" w483 {
                      tunnel: w482 -> [w485 w493 w496 w504]
                      tunnel: w481 -> [w487 w491 w500 w505]
                      tunnel: [w484 w490 w497 w504] -> w480
                      tunnel: [w486 w492 w501 w505] -> w479
                      tunnel: [TRUE ("Cursor.Visible") TRUE ("Cursor.Visible") FALSE ("Cursor.Visible") FALSE ("Cursor.Visible")] -> w478
                      frame "XY" {
                        n215 = Increment(x=w485) -> (x+1=w484:dbl)
                        n216 = Divide(x=w487, y=2.0) -> (x/y=w486:dbl)
                      }
                      frame "XZ" {
                        n217 = Divide(x=w493, y=2.0) -> (x/y=w490:dbl)
                        n218 = Increment(x=w491) -> (x+1=w492:dbl)
                      }
                      frame "XYZ" {
                        n219 = Divide(x=w496, y=2.0) -> (x/y=w497:dbl)
                        n220 = Divide(x=w500, y=2.0) -> (x/y=w501:dbl)
                      }
                      frame "YZ", Default {
                      }
                    }
                  }
                  frame "XYZ" {
                    n221 = case shown="\"YZ\"" w511 {
                      tunnel: w510 -> [w512 w524 w529 w532]
                      tunnel: w509 -> [w516 w519 w526 w533]
                      tunnel: [w513 w523 w528 w532] -> w508
                      tunnel: [w517 w520 w527 w533] -> w507
                      tunnel: [FALSE ("Cursor.Visible") TRUE ("Cursor.Visible") TRUE ("Cursor.Visible") FALSE ("Cursor.Visible")] -> w506
                      frame "XY" {
                        n222 = Divide(x=w512, y=2.0) -> (x/y=w513:dbl)
                        n223 = Divide(x=w516, y=2.0) -> (x/y=w517:dbl)
                      }
                      frame "XZ" {
                        n224 = Divide(x=w524, y=2.0) -> (x/y=w523:dbl)
                        n225 = Increment(x=w519) -> (x+1=w520:dbl)
                      }
                      frame "YZ" {
                        n226 = Increment(x=w529) -> (x+1=w528:dbl)
                        n227 = Divide(x=w526, y=2.0) -> (x/y=w527:dbl)
                      }
                      frame "XYZ", Default {
                      }
                    }
                  }
                }
                n228 = Bundle By Name(cluster=w416, "Last_Scan_Mode"=w414, "Current_Scan_Mode"=w413) -> (w411:T8)
                n229 = property on="Channel 1" class="IntGraph (strict)"("Cursor.Cursor X"=w419, "Cursor.Cursor Y"=w418, "Cursor.Visible"=w417) -> ()  [unwired: 2 in, 2 out]
                n230 = call "Scan Parameters Action Engine.vi"("Action"=enum16{"Read", "Write"}."Write", "Scan Parameters IN"=w411) -> ()  [unwired: 13 in, 1 out]
              }
              frame "Beam Scanning" {
              }
            }
          }
        }
        n231 = case shown="True" w349 {
          tunnel: w351 -> [w389 w397]
          tunnel: [w389 w395] -> w343
          tunnel: w340 -> [_ w394]
          frame False {
          }
          frame True {
            n232 = Unbundle By Name(w397) -> ("Image Dimension (um)"=w391:dbl[], "Image Format"=w401:u16)
            n233 = for {
              tunnel: w394 -> [w402] mode=indexing
              tunnel: w391 -> [w403] mode=indexing
              tunnel: [w403] -> w393
              stop <- w402 stop-if-true
            }
            n234 = Array Size(array=w391) -> (size(s)=w390:i32)
            n235 = To Double Precision Float(number=w401) -> (double precision float=w399:dbl)
            n236 = Initialize Array(w393, w390) -> (w392:dbl[])
            n237 = Divide(x=w392, y=w399) -> (x/y=w400:dbl[])
            n238 = Multiply(x=w400, y=1000.0) -> (x*y=w396:dbl[])
            n239 = Bundle By Name(cluster=w397, "Image Dimension (um)"=w392, "Pixel Size (nm)"=w396) -> (w395:T6)
          }
        }
        n240 = Unbundle By Name(w343) -> ("Image Dimension (um)"=w361:dbl[], "Scan Type"=w366:enum16{"Sample Scanning", "Beam Scanning"})
        n241 = Equal?(x=w366, y=enum16{"Sample Scanning", "Beam Scanning"}."Beam Scanning") -> (x = y?=w344:bool)
        n242 = Index Array(array=w361, index=0) -> (element=w368:dbl)
        n243 = call "Res Mirror um to Volts.vi"("Image Size (um)"=w368) -> ("Voltage (V)"=w369:dbl)
        n244 = Select(t=16110.0, s=w344, f=100.0) -> (s? t:f=w345:dbl)
        n245 = In Range and Coerce(upper limit=4.8, x=w369, lower limit=0.0) -> (coerced(x)=w370:dbl)  [unwired: 1 out]
        n246 = Bundle By Name(cluster=w343, "Fast Axis Frequency (Hz)"=w345) -> (w342:T6)
        n247 = call "Volts to I16.vi"("Voltage (V)"=w370) -> ("I16"=w365:i16)  [unwired: 13 in, 1 out]
        n248 = call "Manual Controls Action Engine.vi"("Action"=enum16{"Read", "Write"}."Read") -> ("Manual Controls Out"=w356:T7)  [unwired: 14 in]
        n249 = Bundle By Name(cluster=w356, "Res Mirror Amp (I16)"=w365, "Res Mirror Mute"=w344) -> (w354:T7)
        n250 = call "Image Aquisition Param Ctrl_AE.vi"("Action"=enum16{"READ", "WRITE"}."WRITE", "Image Acquisition Parameters In"=w342) -> ()  [unwired: 9 in, 1 out]
        n251 = call "FPGA-7842R-Control V1.vi"("Action"=FPGA-7842R-Reference."Set Res Mirror", "Manual Controls"=w354, "Initialize"=TRUE) -> ()  [unwired: 12 in, 1 out]
        n252 = call "Manual Controls Action Engine.vi"("Action"=enum16{"Read", "Write"}."Write", "Manual Controls In"=w354) -> ()  [unwired: 13 in, 1 out]
      }
      event Value Change {
        n253 = event-data() -> ("CtlRef"=w538:refnum<vi>)  [unwired: 1 in, 2 out]
        n254 = property class="Bool"(reference=w538) -> ("Label.Text"=w537:string)  [unwired: 1 in, 2 out]
        n255 = call "Image Aquisition Param Ctrl_AE.vi"("Action"=enum16{"READ", "WRITE"}."READ") -> ("Image Acquisition Parameters Out"=w535:T6)  [unwired: 10 in]
        n256 = case shown="\"SetZoom\", Default" w537 {
          tunnel: w535 -> [w541 w551 w607]
          tunnel: "Focus Control" -> [_ w550 w606]
          frame "SetZoom", Default {
            n257 = control-ref of="Channel 1"() -> (w540:refnum<vi>)
            n258 = call "Set_Focus_Plane.vi"("Image Acquisition Parameters Out"=w541, "IntensityGraph in"=w540) -> ()  [unwired: 10 in]
          }
          frame "ZoomUp" {
            n259 = Unbundle By Name(w550) -> ("ZoomStepI16"=w547:enum16{"Coarse", "Medium", "Fine"})
            n260 = Unbundle By Name(w551) -> ("Scan Type"=w549:enum16{"Sample Scanning", "Beam Scanning"}, "Scan Mode"=w548:enum16{"XY", "XZ", "YZ", "XYZ"})
            n261 = case shown="\"Medium\"" w547 {
              tunnel: [i16 500 i16 150 i16 50] -> w545
              frame "Coarse", Default {
              }
              frame "Medium" {
              }
              frame "Fine" {
              }
            }
            n262 = call "Manual Controls Action Engine.vi"("Action"=enum16{"Read", "Write"}."Read") -> ("Manual Controls Out"=w546:T7)  [unwired: 14 in]
            n263 = case shown="\"Sample Scanning\", Default" w549 {
              tunnel: w548 -> [w565 w591]
              tunnel: w546 -> [w564 w590]
              tunnel: w545 -> [w563 w589]
              tunnel: [w562 w586] -> w544
              frame "Sample Scanning", Default {
                n264 = case shown="\"XZ\"" w565 {
                  tunnel: w564 -> [w570 w575 w580 w585]
                  tunnel: w563 -> [w568 w573 w578 w583]
                  tunnel: [w567 w572 w577 w582] -> w562
                  tunnel: [w566 w571 w576 w581] -> w559
                  frame "XZ" {
                    n265 = Unbundle By Name(w570) -> ("Y Axis Voltage (I16)"=w569:i16)
                    n266 = Add(x=w569, y=w568) -> (x+y=w566:i16)
                    n267 = Bundle By Name(cluster=w570, "Y Axis Voltage (I16)"=w566) -> (w567:T7)
                  }
                  frame "YZ" {
                    n268 = Unbundle By Name(w575) -> ("X Axis Voltage (I16)"=w574:i16)
                    n269 = Add(x=w574, y=w573) -> (x+y=w571:i16)
                    n270 = Bundle By Name(cluster=w575, "X Axis Voltage (I16)"=w571) -> (w572:T7)
                  }
                  frame "XYZ" {
                    n271 = Unbundle By Name(w580) -> ("Z Axis Voltage (I16)"=w579:i16)
                    n272 = Add(x=w579, y=w578) -> (x+y=w576:i16)
                    n273 = Bundle By Name(cluster=w580, "Z Axis Voltage (I16)"=w576) -> (w577:T7)
                  }
                  frame "XY" {
                    n274 = Unbundle By Name(w585) -> ("Z Axis Voltage (I16)"=w584:i16)
                    n275 = Add(x=w584, y=w583) -> (x+y=w581:i16)
                    n276 = Bundle By Name(cluster=w585, "Z Axis Voltage (I16)"=w581) -> (w582:T7)
                  }
                }
                n277 = call "FPGA-7842R-Control V1.vi"("Action"=FPGA-7842R-Reference."Unused Axis I16", "Initialize"=TRUE, "Unused Axis Offset (I16)"=w559) -> ()  [unwired: 12 in, 1 out]
                n278 = call "Scan Parameters Action Engine.vi"("Action"=enum16{"Read", "Write"}."Read") -> ("Scan Parameters OUT"=w558:T8)  [unwired: 14 in]
                n279 = Bundle By Name(cluster=w558, "Unused_Axis_I16"=w559) -> (w557:T8)
                n280 = call "Scan Parameters Action Engine.vi"("Action"=enum16{"Read", "Write"}."Write", "Scan Parameters IN"=w557) -> ()  [unwired: 13 in, 1 out]
              }
              frame "Beam Scanning" {
                n281 = case shown="\"XY\", Default" w591 {
                  tunnel: w590 -> [w596]
                  tunnel: w589 -> [w594]
                  tunnel: [w593] -> w586
                  frame "XY", Default {
                    n282 = Unbundle By Name(w596) -> ("Z Axis Voltage (I16)"=w595:i16)
                    n283 = Add(x=w595, y=w594) -> (x+y=w592:i16)
                    n284 = Bundle By Name(cluster=w596, "Z Axis Voltage (I16)"=w592) -> (w593:T7)
                  }
                }
                n285 = call "FPGA-7842R-Control V1.vi"("Action"=FPGA-7842R-Reference."Stage Control", "Manual Controls"=w586, "Initialize"=TRUE) -> ()  [unwired: 12 in, 1 out]
              }
            }
            n286 = call "Manual Controls Action Engine.vi"("Action"=enum16{"Read", "Write"}."Write", "Manual Controls In"=w544) -> ()  [unwired: 13 in, 1 out]
          }
          frame "ZoomDown" {
            n287 = Unbundle By Name(w607) -> ("Scan Type"=w605:enum16{"Sample Scanning", "Beam Scanning"}, "Scan Mode"=w604:enum16{"XY", "XZ", "YZ", "XYZ"})
            n288 = Unbundle By Name(w606) -> ("ZoomStepI16"=w603:enum16{"Coarse", "Medium", "Fine"})
            n289 = case shown="\"Medium\"" w603 {
              tunnel: [i16 500 i16 150 i16 50] -> w599
              frame "Coarse", Default {
              }
              frame "Medium" {
              }
              frame "Fine" {
              }
            }
            n290 = call "Manual Controls Action Engine.vi"("Action"=enum16{"Read", "Write"}."Read") -> ("Manual Controls Out"=w601:T7)  [unwired: 14 in]
            n291 = Negate(x=w599) -> (-x=w597:i16)
            n292 = case shown="\"Beam Scanning\"" w605 {
              tunnel: w604 -> [w614 w638 _]
              tunnel: w601 -> [w613 w637 w644]
              tunnel: w597 -> [w612 w636 _]
              tunnel: [w611 w635 w644] -> w598
              frame "Sample Scanning" {
                n293 = case shown="\"XZ\"" w614 {
                  tunnel: w613 -> [w619 w624 w629 w634]
                  tunnel: w612 -> [w617 w622 w627 w632]
                  tunnel: [w615 w620 w625 w630] -> w611
                  frame "XZ" {
                    n294 = Unbundle By Name(w619) -> ("Y Axis Voltage (I16)"=w618:i16)
                    n295 = Add(x=w618, y=w617) -> (x+y=w616:i16)
                    n296 = Bundle By Name(cluster=w619, "Y Axis Voltage (I16)"=w616) -> (w615:T7)
                  }
                  frame "YZ" {
                    n297 = Unbundle By Name(w624) -> ("X Axis Voltage (I16)"=w623:i16)
                    n298 = Add(x=w623, y=w622) -> (x+y=w621:i16)
                    n299 = Bundle By Name(cluster=w624, "X Axis Voltage (I16)"=w621) -> (w620:T7)
                  }
                  frame "XYZ" {
                    n300 = Unbundle By Name(w629) -> ("Z Axis Voltage (I16)"=w628:i16)
                    n301 = Add(x=w628, y=w627) -> (x+y=w626:i16)
                    n302 = Bundle By Name(cluster=w629, "Z Axis Voltage (I16)"=w626) -> (w625:T7)
                  }
                  frame "XY" {
                    n303 = Unbundle By Name(w634) -> ("Z Axis Voltage (I16)"=w633:i16)
                    n304 = Add(x=w633, y=w632) -> (x+y=w631:i16)
                    n305 = Bundle By Name(cluster=w634, "Z Axis Voltage (I16)"=w631) -> (w630:T7)
                  }
                }
              }
              frame "Beam Scanning" {
                n306 = case shown="\"XY\", Default" w638 {
                  tunnel: w637 -> [w643]
                  tunnel: w636 -> [w641]
                  tunnel: [w639] -> w635
                  frame "XY", Default {
                    n307 = Unbundle By Name(w643) -> ("Z Axis Voltage (I16)"=w642:i16)
                    n308 = Add(x=w642, y=w641) -> (x+y=w640:i16)
                    n309 = Bundle By Name(cluster=w643, "Z Axis Voltage (I16)"=w640) -> (w639:T7)
                  }
                }
              }
              frame Default {
              }
            }
            n310 = call "Manual Controls Action Engine.vi"("Action"=enum16{"Read", "Write"}."Write", "Manual Controls In"=w598) -> ()  [unwired: 13 in, 1 out]
          }
        }
      }
      event "SLM", "Timing": Value Change {
        n311 = event-data() -> ("CtlRef"=w648:refnum<vi>, "NewVal"=w646:bool)  [unwired: 1 in, 4 out]
        n312 = property class="Bool (strict)"(reference=w648) -> ("Label.Text"=w647:string)  [unwired: 1 in, 2 out]
        n313 = case shown="\"SLM\"" w647 {
          tunnel: w646 -> [_ w649 w665]
          frame "False", Default {
          }
          frame "SLM" {
            n314 = case shown="False" w649 {
              frame False {
                n315 = call "SLM AE.vi"("Action"=enum16{"READ", "WRITE"}."READ") -> ("SLM Ref Out"=w656:refnum<vi>)  [unwired: 10 in]
                n316 = To Variant(anything=TRUE) -> (Variant=w655:variant)
                n317 = invoke class="VI" method="Ctrl Val.Set"(reference=w656, "Control Name"="Exit VI", "Value"=w655) -> (reference out=w652:refnum<vi>, error out=w651:errorcluster)  [unwired: 2 in, 3 out]
                n318 = disable-structure shown="Disabled" {
                  disable-tunnel: w651 -> [w659 _]
                  disable-tunnel: [w658 _] -> w650
                  frame Disabled {
                    n319 = invoke on="Hamamatsu LCOS" class="SubPnl" method="Remove VI"(error in=w659) -> (error out=w658:errorcluster)  [unwired: 2 in, 2 out]
                  }
                  frame Enabled {
                  }
                }
                n320 = Close Reference(reference=w652, error in (no error)=w650) -> ()  [unwired: 1 out]
              }
              frame True {
                n321 = Open VI Reference(vi path=path "C:/Users/STED/Desktop/2014-12-09 Portable_SLM/2014-12-09 Portable_SLM/SLM CONTROL v2.vi") -> (vi reference=w663:refnum<vi>)  [unwired: 5 in, 1 out]
                n322 = invoke class="VI" method="Run VI"(reference=w663, "Wait until done"=FALSE ("Wait Until Done")) -> (reference out=w660:refnum<vi>)  [unwired: 3 in, 4 out]
                n323 = invoke on="Hamamatsu LCOS" class="SubPanel" method="Insert VI"("VI Ref"=w660) -> ()  [unwired: 3 in, 4 out]
                n324 = call "SLM AE.vi"("Action"=enum16{"READ", "WRITE"}."WRITE", "SLM Ref In"=w660) -> ()  [unwired: 9 in, 1 out]
              }
            }
          }
          frame "Timing" {
            n325 = case shown="False" w665 {
              frame False {
                n326 = call "GateDelay AE.vi"("Action"=enum16{"READ", "WRITE"}."READ") -> ("Gate Delay Ref Out"=w672:refnum<vi>)  [unwired: 10 in]
                n327 = To Variant(anything=TRUE) -> (Variant=w671:variant)
                n328 = invoke class="VI" method="Ctrl Val.Set"(reference=w672, "Control Name"="Exit", "Value"=w671) -> (reference out=w667:refnum<vi>, error out=w668:errorcluster)  [unwired: 2 in, 3 out]
                n329 = invoke on="Timing" class="SubPnl" method="Remove VI"(error in=w668) -> (error out=w666:errorcluster)  [unwired: 2 in, 2 out]
                n330 = Close Reference(reference=w667, error in (no error)=w666) -> ()  [unwired: 1 out]
              }
              frame True {
                n331 = Open VI Reference(vi path=path "C:/Users/STED/Documents/STED VIs/Gate Delay Board/DElay Board Test.vi") -> (vi reference=w677:refnum<vi>)  [unwired: 5 in, 1 out]
                n332 = invoke class="VI" method="Run VI"(reference=w677, "Wait until done"=FALSE ("Wait Until Done")) -> (reference out=w674:refnum<vi>)  [unwired: 3 in, 4 out]
                n333 = invoke on="Timing" class="SubPanel" method="Insert VI"("VI Ref"=w674) -> ()  [unwired: 3 in, 4 out]
                n334 = call "GateDelay AE.vi"("Action"=enum16{"READ", "WRITE"}."WRITE", "Gate Delay Ref In"=w674) -> ()  [unwired: 9 in, 1 out]
              }
            }
          }
        }
      }
    }
  }
  n335 = while {
    shift-right: [w687] -> _
    shift-left: "Idle" -> [w688]
    tunnel: w30 -> [w684]
    shift-right: [w682] -> _
    shift-left: w27 -> [w683]
    stop <- w686 stop-if-true
    n336 = call "Image Aquisition Param Ctrl_AE.vi"("Action"=enum16{"READ", "WRITE"}."READ") -> ("Image Acquisition Parameters Out"=w680:T6)  [unwired: 10 in]
    n337 = case shown="\"Start Waveforms\"" w688 {
      selector: w688 -> [_ _ _ w720 _ _ _ _ _ _]
      tunnel: ["Exit" w697 "Idle" ("name (unnamed)") "Arange Displays" ("name (unnamed)") "Start FPGA Acquisition" ("name (unnamed)") "Display" ("name (unnamed)") "Close Images" ("name (unnamed)") "Idle" "Stop Waveforms" ("name (unnamed)") "Start Waveforms" ("name (unnamed)")] -> w687
      tunnel: [TRUE w699 w706 w728 w743 w755 w796 w829 w834 w840] -> w686
      tunnel: FALSE -> [_ w699 w706 w728 w743 w755 w796 w829 w834 w840]
      tunnel: w684 -> [_ w698 _ _ _ _ _ _ _ _]
      tunnel: w683 -> [w693 w696 w707 w726 w740 w753 w794 w827 w835 w841]
      tunnel: [w692 w696 w707 w726 w740 w749 w794 w826 w835 w841] -> w682
      tunnel: w680 -> [_ _ _ w719 _ w748 _ _ _ w838]
      tunnel: "Detectors" -> [_ _ _ w718 _ _ _ _ _ w836]
      frame "Exit" {
        n338 = call "Graph Ref AE.vi"("Action"=enum16{"READ", "WRITE"}."READ") -> ("Graph Ref Out"=w690:refnum<vi>[])  [unwired: 10 in]
        n339 = call "FPGA-7842R-Control V1.vi"("Action"=FPGA-7842R-Reference."Close FPGA", "Initialize"=w693) -> ("Initalized"=w692:bool)  [unwired: 13 in]
        n340 = Close Reference(reference=w690) -> ()  [unwired: 1 in, 1 out]
      }
      frame "Idle", Default {
        n341 = Dequeue Element(queue=w698, timeout in ms (-1)=-1) -> (element=w697:string)  [unwired: 1 in, 3 out]
      }
      frame "Close Images" {
        w702 = u16 0 items=["Read", "Write"] ("Mode")
        w703 = u16 0 items=["Write", "Read"] ("Mode")
        n342 = call "File Action V1.vi"("Mode"=w702) -> ("Files Open"=w701:bool)  [unwired: 12 in, 2 out]
        n343 = call "Image_Actions_V1.vi"("Mode"=w703, "Action"="Trash Images") -> ()  [unwired: 12 in, 2 out]
        n344 = case shown="True" w701 {
          frame False {
          }
          frame True {
            w709 = u16 1 items=["Read", "Write"] ("Mode")
            n345 = call "File Action V1.vi"("Action"="Close Files", "Mode"=w709) -> ()  [unwired: 11 in, 3 out]
          }
        }
      }
      frame "Capture", "Live" {
        w724 = u16 0 items=["Write", "Read"] ("Mode")
        n346 = Cluster To Array(cluster=w718) -> (array=w716:bool[])
        n347 = Index Array(array=w716, index=4) -> (element=w713:bool)
        n348 = Boolean To (0,1)(Boolean=w716) -> (0, 1=w717:i16[])
        n349 = Add Array Elements(numeric array=w717) -> (sum=w714:i16)
        n350 = To Long Integer(number=w714) -> (32bit integer=w711:i32)
        n351 = Unbundle By Name(w719) -> ("Image Format"=w721:u16)
        n352 = Select(t=1, s=w713, f=w711) -> (s? t:f=w710:i32)
        n353 = case shown="\"Capture\"" w720 {
          tunnel: w719 -> [_ w730]
          tunnel: w710 -> [_ w729]
          frame Default {
          }
          frame "Capture" {
            w733 = u16 1 items=["Read", "Write"] ("Mode")
            n354 = call "File Action V1.vi"("Action"="Open Files", "Mode"=w733, "Image Acquisition Parameters"=w730, "File Path IN"="Save File Path", "Number of Channels"=w729) -> ("File Path OUT"=w731:path)  [unwired: 8 in, 2 out]
            n355 = local write "Save File Path"(w731) -> ()
          }
        }
        n356 = To Long Integer(number=w721) -> (32bit integer=w723:i32)
        n357 = Bundle(w723, w723) -> (w722:cluster{i32, i32})  [unwired: 1 in]
        n358 = call "Image_Actions_V1.vi"("Image Size (Pixels)"=w722, "Mode"=w724, "Number of Channels"=w710, "Action"="Create Images") -> ()  [unwired: 10 in, 2 out]
      }
      frame "Arange Displays" {
        w738 = u16 1 items=["Write", "Read"] ("Mode")
        w742 = 1.0  # Aspect Ratio (h/w)
        w741 = u16 1 items=["Read", "Write"] ("Action")
        n359 = call "Graph Ref AE.vi"("Action"=enum16{"READ", "WRITE"}."READ") -> ("Graph Ref Out"=w735:refnum<vi>[])  [unwired: 10 in]
        n360 = call "Image_Actions_V1.vi"("Mode"=w738) -> ("Image REFs OUT"=w739:T19[])  [unwired: 13 in, 1 out]
        n361 = Array Size(array=w739) -> (size(s)=w737:i32)
        n362 = call "Arange_Displays_V2.vi"("Display References"=w735, "Action"=w741, "Number of Channels"=w737, "Aspect Ratio (h/w)"=w742) -> ()  [unwired: 11 in, 1 out]
      }
      frame "Start Waveforms" {
        n363 = call "Initialize Waveforms V4.vi"("Image Acquisition Parameters"=w748) -> ("Waveform Data to FPGA"=w754:T20)  [unwired: 14 in]
        n364 = Unbundle By Name(w748) -> ("Scan Type"=w747:enum16{"Sample Scanning", "Beam Scanning"})
        n365 = call "FPGA-7842R-Control V1.vi"("Waveform Data"=w754, "Action"=FPGA-7842R-Reference."Start Waveforms", "Image Acquisition Parameters"=w748, "Initialize"=w753) -> ("Initalized"=w750:bool)  [unwired: 11 in]
        n366 = Equal?(x=w747, y=enum16{"Sample Scanning", "Beam Scanning"}."Sample Scanning" ("Scan Type")) -> (x = y?=w745:bool)
        n367 = case shown="True" w745 {
          tunnel: w750 -> [w756 w761]
          tunnel: [w756 w760] -> w749
          frame False {
          }
          frame True {
            n368 = call "Scan Parameters Action Engine.vi"("Action"=enum16{"Read", "Write"}."Read") -> ("Scan Parameters OUT"=w758:T8)  [unwired: 14 in]
            n369 = Unbundle By Name(w758) -> ("Unused_Axis_I16"=w757:i16)
            n370 = call "FPGA-7842R-Control V1.vi"("Action"=FPGA-7842R-Reference."Unused Axis I16", "Initialize"=w761, "Unused Axis Offset (I16)"=w757) -> ("Initalized"=w760:bool)  [unwired: 12 in]
          }
        }
      }
      frame "Display" {
        w788 = u16 1 items=["Write", "Read"] ("Mode")
        n371 = call "Image_Actions_V1.vi"("Mode"=w788) -> ("Image REFs OUT"=w790:T19[])  [unwired: 13 in, 1 out]
        n372 = Array Size(array=w790) -> (size(s)=w786:i32)
        n373 = Decrement(x=w786) -> (x-1=w785:i32)
        n374 = for {
          N: 6 -> [_]
          tunnel: w785 -> [w824]
          tunnel: [w822] -> w789 mode=indexing
          i -> [w823]
          n375 = Greater Or Equal?(x=w824, y=w823) -> (x >= y?=w822:bool)
        }
        n376 = Obtain Notifier(name (unnamed)="Running", notification data type=FALSE) -> (notifier out=w793:refnum<notifier>)  [unwired: 2 in, 2 out]
        n377 = Index Array(array=w789, index #1=1 ("index"), index #2=2 ("index"), index #3=3 ("index"), index #4=4 ("index"), index #5=5 ("index")) -> (element #1=w774:bool, element #2=w773:bool, element #3=w772:bool, element #4=w771:bool, element #5=w770:bool)
        n378 = Index Array(array=w790, index #1=0 ("index"), index #2=1 ("index"), index #3=2 ("index"), index #4=3 ("index"), index #5=4 ("index"), index #6=5 ("index")) -> (element #1=w769:T19, element #2=w768:T19, element #3=w767:T19, element #4=w766:T19, element #5=w765:T19, element #6=w764:T19)
        n379 = while {
          tunnel: w774 -> [w811]
          tunnel: w773 -> [w810]
          tunnel: w772 -> [w806]
          tunnel: w771 -> [w803]
          tunnel: w770 -> [w802]
          tunnel: w769 -> [w809]
          tunnel: w768 -> [w808]
          tunnel: w767 -> [w807]
          tunnel: w766 -> [w805]
          tunnel: w765 -> [w799]
          tunnel: w764 -> [w804]
          tunnel: w793 -> [w801]
          stop <- w800 stop-if-true
          n380 = Get Notifier Status(notifier=w801) -> (current notification=w800:bool)  [unwired: 1 in, 4 out]
          n381 = case shown="False" w811 {
            tunnel: w808 -> [_ w821]
            frame False {
            }
            frame True {
              n382 = call "IMAQ ImageToArray"("Image"=w821) -> ("Image Pixels (Float)"=→"Channel 2":sgl[][])  [unwired: 3 in, 4 out]
            }
          }
          n383 = case shown="False" w810 {
            tunnel: w807 -> [_ w819]
            frame False {
            }
            frame True {
              n384 = call "IMAQ ImageToArray"("Image"=w819) -> ("Image Pixels (Float)"=→"Channel 3":sgl[][])  [unwired: 3 in, 4 out]
            }
          }
          n385 = call "IMAQ ImageToArray"("Image"=w809) -> ("Image Pixels (Float)"=→"Channel 1":sgl[][])  [unwired: 3 in, 4 out]
          n386 = Wait (ms)(milliseconds to wait=u32 30) -> ()  [unwired: 1 out]
          n387 = case shown="False" w806 {
            tunnel: w805 -> [_ w817]
            frame False {
            }
            frame True {
              n388 = call "IMAQ ImageToArray"("Image"=w817) -> ("Image Pixels (Float)"=→"Channel 4":sgl[][])  [unwired: 3 in, 4 out]
            }
          }
          n389 = case shown="False" w803 {
            tunnel: w799 -> [_ w815]
            frame False {
            }
            frame True {
              n390 = call "IMAQ ImageToArray"("Image"=w815) -> ("Image Pixels (Float)"=→"Channel 5":sgl[][])  [unwired: 3 in, 4 out]
            }
          }
          n391 = case shown="False" w802 {
            tunnel: w804 -> [_ w813]
            frame False {
            }
            frame True {
              n392 = call "IMAQ ImageToArray"("Image"=w813) -> ("Image Pixels (Float)"=→"Channel 6":sgl[][])  [unwired: 3 in, 4 out]
            }
          }
        }
      }
      frame "Stop Waveforms" {
        n393 = call "FPGA-7842R-Control V1.vi"("Action"=FPGA-7842R-Reference."Stop Waveforms", "Initialize"=w827) -> ("Initalized"=w826:bool)  [unwired: 13 in]
      }
      frame "Stop Acquisition" {
        n394 = call "FPGA-7842R-Control V1.vi"("Action"=FPGA-7842R-Reference."Laser Control", "Laser Controls"=T5 {"STED Power (V)"=0.0, "590 Power (V)"=0.0, "STED"=FALSE, "640 nm"=FALSE, "590 nm"=FALSE, "485 nm"=FALSE, "Manual Control"=FALSE} ("Laser Controls 2"), "Initialize"=TRUE) -> ()  [unwired: 12 in, 1 out]
      }
      frame "Start FPGA Acquisition" {
        n395 = Unbundle By Name(w838) -> ("Scan Type"=w837:enum16{"Sample Scanning", "Beam Scanning"})
        n396 = case shown="\"Sample Scanning\", Default" w837 {
          tunnel: w838 -> [w843 w851]
          tunnel: w836 -> [w842 w849]
          frame "Sample Scanning", Default {
            n397 = vi-ref "FPGA Sample Scanning V1.vi"() -> (w846:refnum<vi>)
            n398 = property class="VI Interface Type 0"(reference=w846) -> ("Path"=w844:path)  [unwired: 1 in, 2 out]
            n399 = Open VI Reference(type specifier VI Refnum (for type only)=w846, vi path=w844, options=128) -> (vi reference=w847:refnum<vi>)  [unwired: 3 in, 1 out]
            n400 = call-by-ref "Start Asynchronous Call"(reference=w847, "Detectors"=w842, "Image Acquisition Parameters"=w843) -> (reference out=w848:refnum<vi>)  [unwired: 2 in, 1 out]
            n401 = Close Reference(reference=w848) -> ()  [unwired: 1 in, 1 out]
          }
          frame "Beam Scanning" {
            n402 = vi-ref "FPGA Beam Scanning V1.vi"() -> (w854:refnum<vi>)
            n403 = property class="VI Interface Type 0"(reference=w854) -> ("Path"=w852:path)  [unwired: 1 in, 2 out]
            n404 = Open VI Reference(type specifier VI Refnum (for type only)=w854, vi path=w852, options=128) -> (vi reference=w850:refnum<vi>)  [unwired: 3 in, 1 out]
            n405 = call-by-ref "Start Asynchronous Call"(reference=w850, "Detectors"=w849, "Image Acquisition Parameters"=w851) -> (reference out=w855:refnum<vi>)  [unwired: 2 in, 1 out]
            n406 = Close Reference(reference=w855) -> ()  [unwired: 1 in, 1 out]
          }
        }
      }
    }
  }
